vi "GetHeader.vi"(7 "error in":errorcluster, 10 "refnum in":refnum<file>) -> (0 "error out":errorcluster, 2 "Header":T1, 3 "refnum out":refnum<file>)   [LabVIEW 2012]
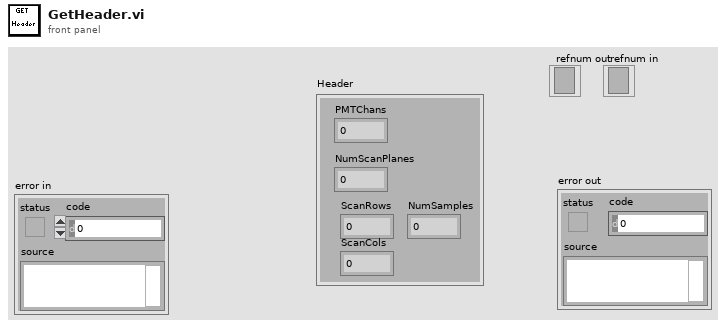
[diagram p1: front panel]
types:
  T1 = cluster{"PMTChans":i32, "NumScanPlanes":i32, "ScanRows":i32, "ScanCols":i32, "NumSamples":i32}
  T2 = enum16{"big-endian, network order", "native, host order", "little-endian"}
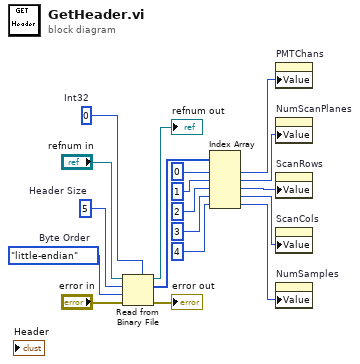
[diagram p0: block diagram]
diagram:
  w17 = 5  # Header Size
  w18 = T2."little-endian"  # Byte Order
  w14 = 0  # Int32
  n1 = Read from Binary File(5:w14, 8:"error in", 9:w18, 10:w17, 11:"refnum in") -> (0:→"error out":errorcluster, 2:w8:i32[], 3:→"refnum out":refnum<file>)  [unwired: 1 in, 1 out]
  n2 = Index Array(array=w8, index #1=0 ("index"), index #2=1 ("index"), index #3=2 ("index"), index #4=3 ("index"), index #5=4 ("index")) -> (element #1=w7:i32, element #2=w6:i32, element #3=w5:i32, element #4=w4:i32, element #5=w3:i32)
  n3 = property on="PMTChans" class="DigNum (strict)"("Value"=w7) -> ()  [unwired: 2 in, 2 out]
  n4 = property on="NumScanPlanes" class="DigNum (strict)"("Value"=w6) -> ()  [unwired: 2 in, 2 out]
  n5 = property on="ScanRows" class="DigNum (strict)"("Value"=w5) -> ()  [unwired: 2 in, 2 out]
  n6 = property on="ScanCols" class="DigNum (strict)"("Value"=w4) -> ()  [unwired: 2 in, 2 out]
  n7 = property on="NumSamples" class="DigNum (strict)"("Value"=w3) -> ()  [unwired: 2 in, 2 out]
